vi "helper-collect-wind-speed.vi"(8 "error in":errorcluster, 11 "Value in":dbl) -> (0 "error out":errorcluster, 1 "_W_DIR_BUF Node":T1={"ADDR"=0, "Label"="", "Type"=enum."DI", "Mode"=enum."RIO", "Value"="", "Tags"="", "calibration"=[]} {"calibration"."Y" format="%#.3f"; "calibration"."X" format="%#.3f"; "ADDR" format="%04d"}, 2 "_W_DIR Node":T1={"ADDR"=0, "Label"="", "Type"=enum."DI", "Mode"=enum."RIO", "Value"="", "Tags"="", "calibration"=[]} {"calibration"."Y" format="%#.3f"; "calibration"."X" format="%#.3f"; "ADDR" format="%04d"}, 3 "Result":dbl)   [LabVIEW 2024]
uses:
  controls/IONode.ctl
  controls/type.address.ctl
  controls/enum.io.type.ctl
  controls/enum.io.mode.ctl
  controls/typeXyPoint.ctl
  controls/enumVarCtrlIO.ctl
  <vilib>/Utility/error.llb/Trim Whitespace.vi
  <vilib>/Utility/error.llb/Trim Whitespace One-Sided.vi
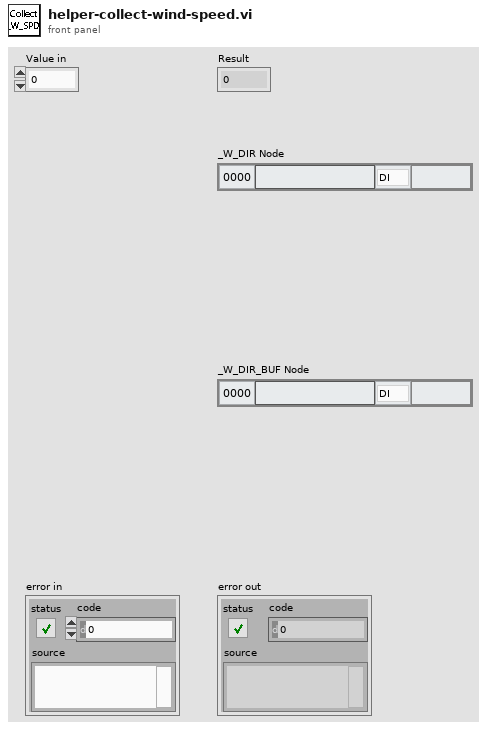
[diagram p1: front panel]
types:
  T1 = typedef "IONode.ctl" = cluster{"ADDR":T2, "Label":string, "Type":T3, "Mode":T4, "Value":string, "Tags":string, "calibration":T5[]}
  T2 = typedef "type.address.ctl" = u16
  T3 = typedef "enum.io.type.ctl" = enum16{"Type", "DI", "DO", "AI", "AO", "VL", "BUF"}
  T4 = typedef "enum.io.mode.ctl" = enum16{"Mode", "RIO", "SIM"}
  T5 = typedef "typeXyPoint.ctl" = cluster{"X":dbl, "Y":dbl}
  T6 = typedef "enumVarCtrlIO.ctl" = enum16{"IO Get By Key", "IO List Configs", "IO Add By Key", "IO Modify Value By Key", "IO Modify Calib By Key", "IO Modify ADDR By Key", "IO Modify Mode By Key", "IO Modify Type By Key", "IO Modify Name By Key", "IO Remove By Key", "IO Remove All"}
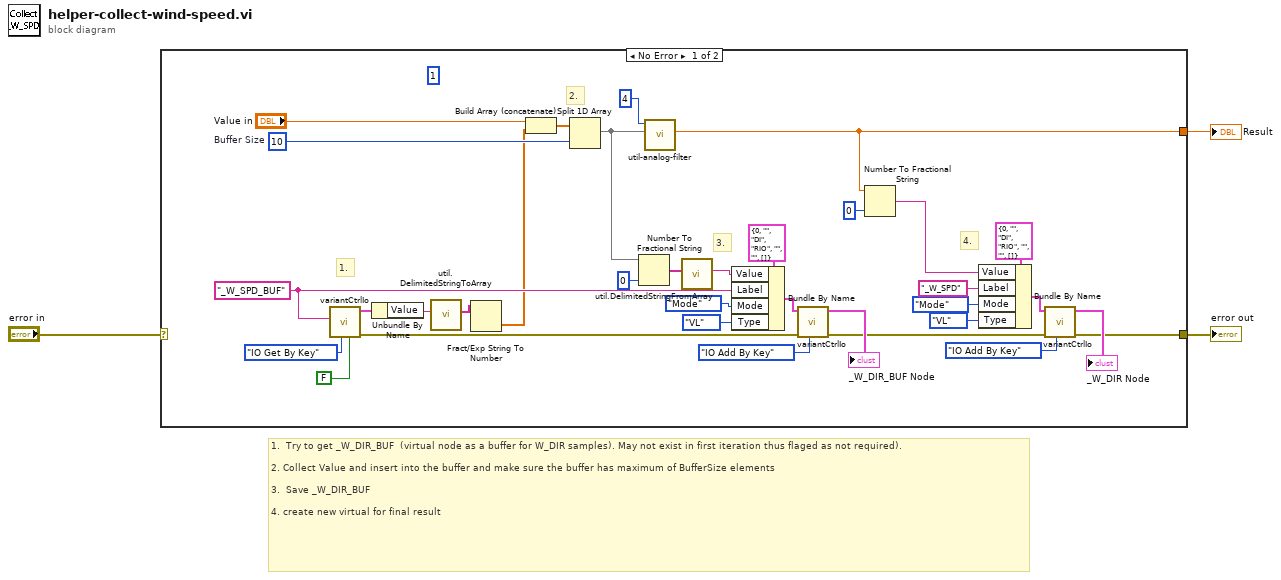
[diagram p0: block diagram]
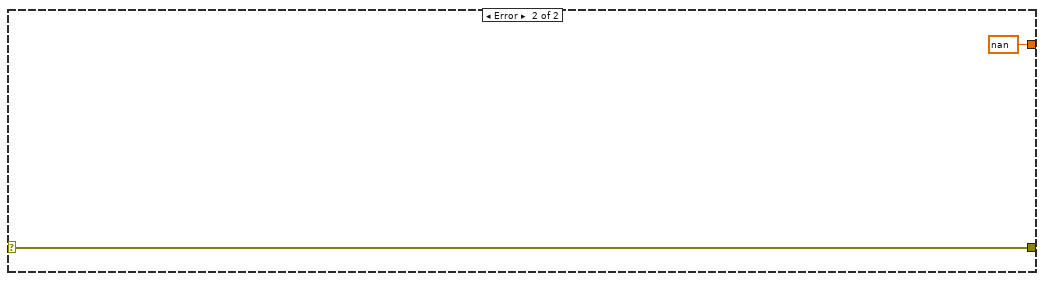
[diagram p2: hidden frame]
diagram:
  # "1.  Try to get _W_DIR_BUF  (virtual node as a buffer for W_DIR samples). May not exist in first iteration thus flaged as not required).\n\n2. Collect Value and insert into the buffer and make sure the buffer has maximum of BufferSize elements\n\n3.  Save _W_DIR_BUF\n\n4. create new virtual for final result"
  n1 = case shown="No Error" "error in" {
    selector: "error in" -> [_ w39]
    tunnel: [w11 w39] -> w3
    tunnel: [w5 nan ("Filtered Value")] -> w1
    frame No Error {
      w24 = "_W_SPD_BUF" ("RecFilename.*")
      w37 = 10  # Buffer Size
      (unwired) i16 1 ("precision (6)")
      # "4."
      # "3."
      # "2."
      # "1."
      n2 = call "variantCtrlIo.vi"("isRequired (T)"=FALSE, "menu (Get Param)"=enumVarCtrlIO."IO Get By Key", "Key (use IOnode Label if empty )"=w24) -> ("error out"=w31:errorcluster, "IOnode out"=w36:T1)  [unwired: 4 in, 3 out]
      n3 = Unbundle By Name(w36) -> ("Value"=w35:string)
      n4 = call "util.DelimitedStringToArray.vi"("delimitaed string"=w35) -> ("array out"=w10:string[])  [unwired: 10 in]
      n5 = Fract/Exp String To Number(string=w10) -> (number=w8:dbl[])  [unwired: 3 in, 1 out]
      n6 = Build Array (concatenate)("Value in", w8) -> (w33:dbl[])
      n7 = Split 1D Array(array=w33, index=w37) -> (first subarray=w7:dbl[])  [unwired: 1 out]
      n8 = Number To Fractional String(number=w7, precision (6)=i16 0) -> (F-format string=w6:string[])  [unwired: 2 in]
      n9 = call "util-analog-filter.vi"("Array"=w7, "# of mins&maxs to remove"=4) -> ("Filtered Value"=w5:dbl)  [unwired: 9 in]
      n10 = call "util.DelimitedStringFromArray.vi"("params array in"=w6) -> ("delimited string out"=w28:string)  [unwired: 10 in]
      n11 = Bundle By Name(cluster=T1 {"ADDR"=0, "Label"="", "Type"=enum."DI", "Mode"=enum."RIO", "Value"="", "Tags"="", "calibration"=[]} ("IoConf in"), "Value"=w28, "Label"=w24, "Mode"=enum.io.mode."Mode", "Type"=enum.io.type."VL" ("type")) -> (w27:T1)
      n12 = call "variantCtrlIo.vi"("menu (Get Param)"=enumVarCtrlIO."IO Add By Key" ("menu in (get)"), "error in"=w31, "IOnode in"=w27) -> ("error out"=w12:errorcluster, "IOnode out"=→"_W_DIR_BUF Node":T1)  [unwired: 4 in, 3 out]
      n13 = Number To Fractional String(number=w5, precision (6)=i16 0) -> (F-format string=w14:string)  [unwired: 2 in]
      n14 = Bundle By Name(cluster=T1 {"ADDR"=0, "Label"="", "Type"=enum."DI", "Mode"=enum."RIO", "Value"="", "Tags"="", "calibration"=[]} ("IoConf in"), "Value"=w14, "Label"="_W_SPD" ("RecFilename.*"), "Mode"=enum.io.mode."Mode", "Type"=enum.io.type."VL" ("type")) -> (w18:T1)
      n15 = call "variantCtrlIo.vi"("menu (Get Param)"=enumVarCtrlIO."IO Add By Key" ("menu in (get)"), "error in"=w12, "IOnode in"=w18) -> ("error out"=w11:errorcluster, "IOnode out"=→"_W_DIR Node":T1)  [unwired: 4 in, 3 out]
    }
    frame Error {
    }
  }
  "error out" <- w3
  "Result" <- w1
